vi "Read Multi Eval Meas EVM Peak Results.vi"(8 "error in (no error)":errorcluster, 9 "Result Type (Current)":i32(ring) items=["Current"=0, "Average"=1, "Maximum"=4], 10 "Instance (1)":T1=1, 11 "VISA resource name":refnum<visa-resource-name>) -> (0 "error out":errorcluster, 1 "EVM Results":cluster{"Low Window":dbl, "High Window":dbl}[](array[cluster]) {"High Window" format="%^.3e"; "Low Window" format="%^.3e"}, 2 "Reliability":i32, 3 "VISA resource name out":refnum<visa-resource-name>)   [LabVIEW 2020, in "Rohde&Schwarz CMWXP NR FR1 Measurement.lvlib"]
doc: "Returns the values of the EVM peak bar graphs for the OFDM symbols in the measured slot. The results of the current, average and maximum bar graphs can be retrieved.\n\nThere is one pair of EVM values per OFDM symbol, for low and high EVM window position respectively.\n\nAttributes:\nRSCMWXPNRFR1M_ATTR_READ_MULTI_EVAL_MEAS_EVM_PEAK_CURRENT_RESULTS\nRSCMWXPNRFR1M_ATTR_READ_MULTI_EVAL_MEAS_EVM_PEAK_AVERAGE_RESULTS\nRSCMWXPNRFR1M_ATTR_READ_MULTI_EVAL_MEAS_EVM_PEAK_MAXIMUM_RESULTS\n\nRemote-control commands:\nREAD:NRSub:MEAS<i>:MEValuation:EVMagnitude:PEAK:CURRent?\nREAD:NRSub:MEAS<i>:MEValuation:EVMagnitude:PEAK:AVERage?\nREAD:NRSub:MEAS<i>:MEValuation:EVMagnitude:PEAK:MAXimum?"
uses:
  <instrlib>/Rohde&Schwarz CMWXP NR FR1 Measurement/Rohde&Schwarz CMWXP NR FR1 Measurement.lvlib
  <instrlib>/Rohde&Schwarz CMWXP NR FR1 Measurement/Private/_Instance.ctl
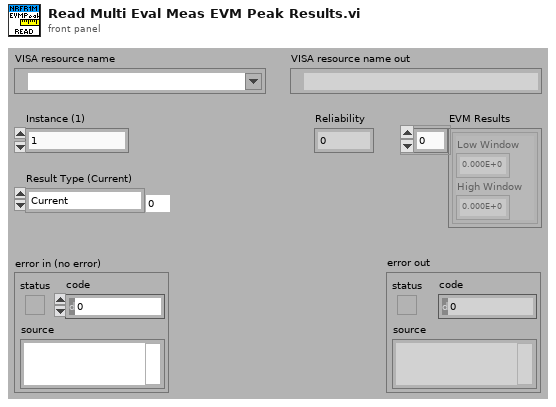
[diagram p1: front panel]
types:
  T1 = typedef "Rohde&Schwarz CMWXP NR FR1 Measurement.lvlib/_Instance.ctl" = i32
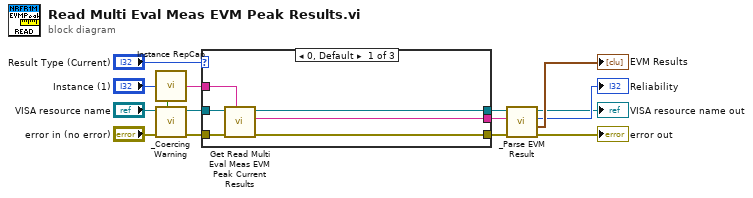
[diagram p0: block diagram]
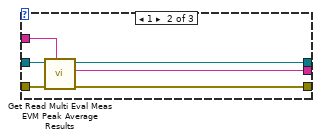
[diagram p2: hidden frame]
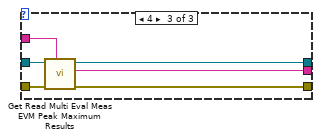
[diagram p3: hidden frame]
diagram:
  n1 = call <instrlib>:"Instance RepCap.vi"("Instance In"="Instance (1)") -> ("In Range?"=w15:bool, "RepCap Identifier Out"=w8:string)  [unwired: 1 in]
  n2 = call <instrlib>:"_Coercing Warning.vi"("In Range?"=w15, "error in (no error)"="error in (no error)", "VISA resource name"="VISA resource name") -> ("error out"=w13:errorcluster, "VISA resource name out"=w14:refnum<visa-resource-name>)  [unwired: 7 in]
  n3 = case shown="0, Default" "Result Type (Current)" {
    tunnel: w14 -> [w21 w27 w33]
    tunnel: w13 -> [w20 w26 w32]
    tunnel: [w19 w25 w31] -> w10
    tunnel: [w18 w24 w30] -> w11
    tunnel: [w17 w23 w29] -> w12
    tunnel: w8 -> [w16 w22 w28]
    frame 0, Default {
      n4 = call "Get Read Multi Eval Meas EVM Peak Current Results"("Repeated Capabilities"=w16, "error in (no error)"=w20, "instrument handle"=w21) -> ("error out"=w17:errorcluster, "Read Multi Eval Meas EVM Peak Current Results"=w18:string, "instrument handle out"=w19:refnum<visa-resource-name>)  [unwired: 6 in]
    }
    frame 1 {
      n5 = call "Get Read Multi Eval Meas EVM Peak Average Results"("Repeated Capabilities"=w22, "error in (no error)"=w26, "instrument handle"=w27) -> ("error out"=w23:errorcluster, "Read Multi Eval Meas EVM Peak Average Results"=w24:string, "instrument handle out"=w25:refnum<visa-resource-name>)  [unwired: 6 in]
    }
    frame 4 {
      n6 = call "Get Read Multi Eval Meas EVM Peak Maximum Results"("Repeated Capabilities"=w28, "error in (no error)"=w32, "instrument handle"=w33) -> ("error out"=w29:errorcluster, "Read Multi Eval Meas EVM Peak Maximum Results"=w30:string, "instrument handle out"=w31:refnum<visa-resource-name>)  [unwired: 6 in]
    }
  }
  n7 = call <instrlib>:"_Parse EVM Result.vi"("error in (no error)"=w12, "Input String"=w11, "VISA resource name"=w10) -> ("error out"=→"error out":errorcluster, "EVM Results"=→"EVM Results":cluster{"Low Window":dbl, "High Window":dbl}[], "Reliability"=→"Reliability":i32, "VISA resource name out"=→"VISA resource name out":refnum<visa-resource-name>)  [unwired: 5 in]
